vi "DAQ_Thermo_SUB_VI.vi"(11 "task in":refnum<k21>="DAQ_3") -> (3 "channel":T1)   [LabVIEW 2022 SP3]
doc: "Tager daq data ind og outputter det på en måde som kan styre et loop"
uses:
  <extravilib>/ChannelInstances/Stream-a[.](dbl)/)Channel.ctl
  <vilib>/DAQmx/read.llb/DAQmx Read (Analog 1D DBL NChan 1Samp).vi
  <extravilib>/ChannelInstances/Stream-a[.](dbl)/Write With Abort.vi
  <extravilib>/ChannelInstances/Stream-a[.](dbl)/Endpoint.vi
  <vilib>/DAQmx/miscellaneous.llb/DAQmx Fill In Error Info.vi
  <extravilib>/ChannelInstances/Stream-a[.](dbl)/)Channel.vi
  <resource>/ChannelSupport/_ChannelSupport/WaitIfNeeded.vi
  <extravilib>/ChannelInstances/Stream-a[.](dbl).lvlib
panel:
  in  "stop":bool
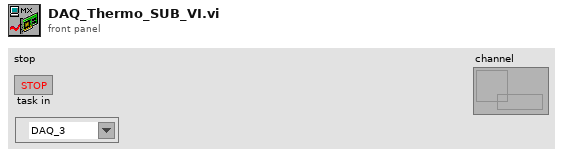
[diagram p1: front panel]
types:
  T1 = typedef "Stream-a[.](dbl).lvlib/)Channel.ctl" = refnum<queue>
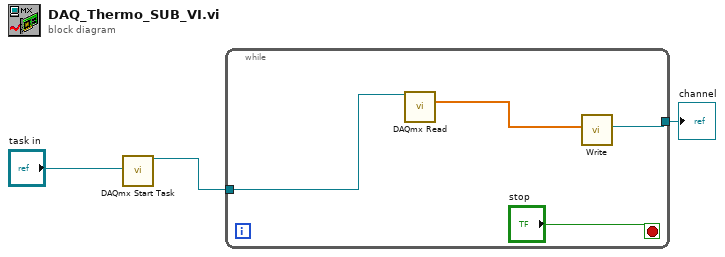
[diagram p0: block diagram]
diagram:
  n1 = call <vilib>:"DAQmx Start Task.vi"("task/channels in"="task in") -> ("task out"=w3:refnum<k21>)  [unwired: 13 in, 1 out]
  n2 = while {
    tunnel: w3 -> [w7]
    tunnel: [w4] -> w1
    stop <- "stop" stop-if-true
    n3 = call-poly <vilib>:"DAQmx Read.vi"("task/channels in"=w7) -> ("data"=w5:dbl[])  [unwired: 12 in, 2 out]
    n4 = call <extravilib>:"Write.vi"("element"=w5) -> ("channel"=w4:T1)  [unwired: 8 in, 2 out]
  }
  "channel" <- w1
